vi "AoA Detection 1st TX Ref Signal.vi"() -> ()   [LabVIEW 2015]
doc: "Continuously generates a communication signal that starts immediately. The device is not synchronized to external reference clocks or time bases."
uses:
  <instrlib>/niUSRP/niUSRP Write Tx Data (CDB Cluster).vi
  <vilib>/measure/NI_MABase.lvlib
panel:
  out "TX1":bool
  out "coerced gain":dbl format="%#_6f"
  in  "active antenna":string="TX1"
  out "coerced carrier frequency":dbl format="%#_6p"
  out "coerced IQ rate":dbl format="%#_6p"
  in  "gain":dbl=10.0 format="%#_6f"
  in  "carrier frequency":dbl=900000000.0 format="%#_6p"
  in  "IQ rate":dbl=1000000.0 format="%#_6p"
  out "TX2":bool
  in  "device names":refnum<k15>="192.168.10.2"
  in  "tone frequency":dbl=10000.0 format="%#_6p"
  out "Waveform Graph":waveform(dbl)[](graph)
  in  "waveform size":dbl=10000.0
  in  "timeout":dbl=10.0
  out "error out":errorcluster
  in  "stop":bool
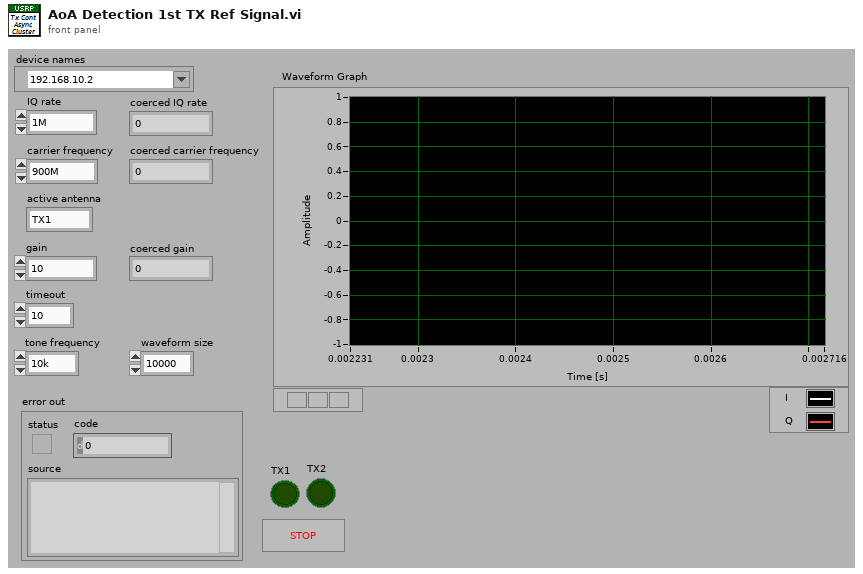
[diagram p1: front panel]
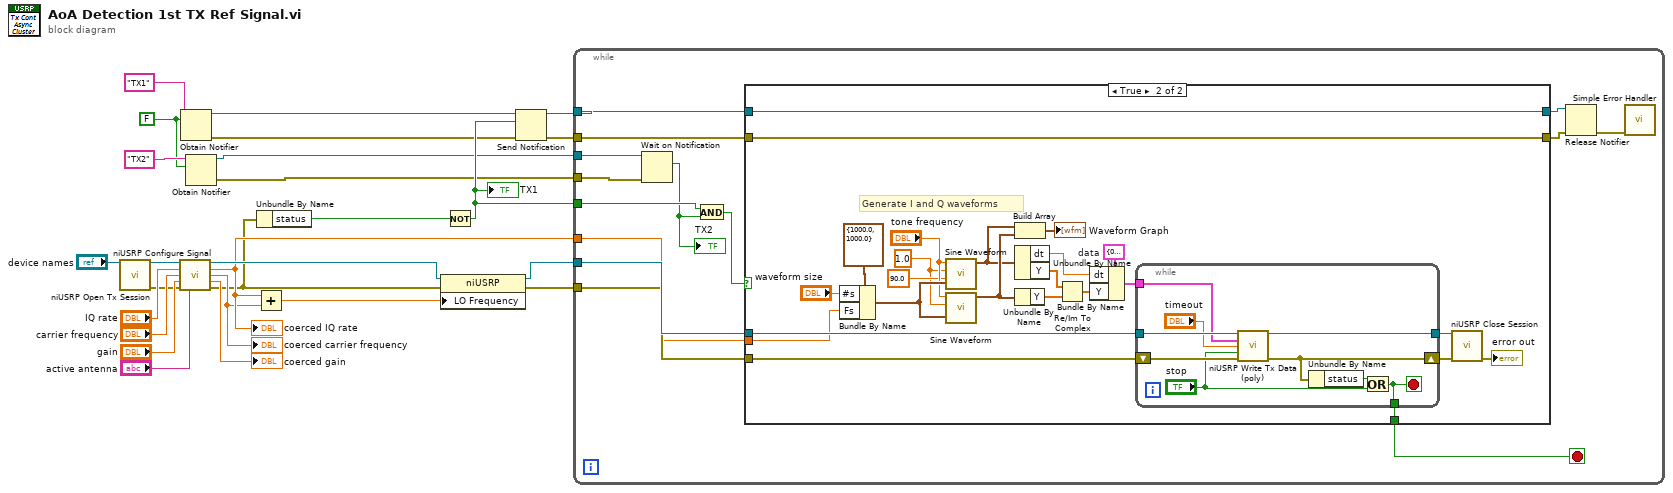
[diagram p0: block diagram]
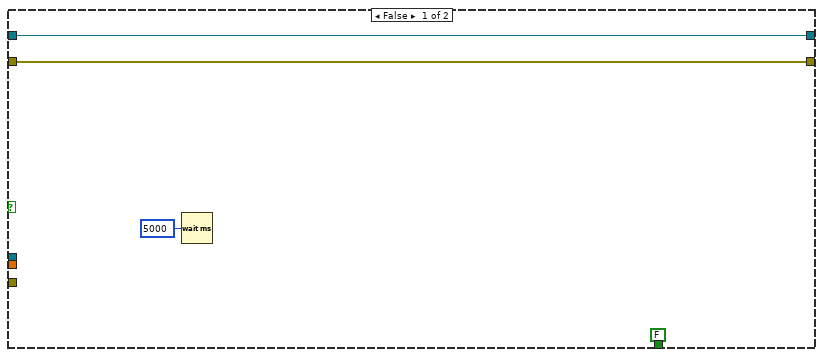
[diagram p2: hidden frame]
diagram:
  w1 = FALSE
  n1 = call <instrlib>:"niUSRP Open Tx Session.vi"("device names"="device names") -> ("session handle out"=w20:refnum<k15>, "error out"=w19:errorcluster)  [unwired: 13 in]
  n2 = call <instrlib>:"niUSRP Configure Signal.vi"("session handle"=w20, "IQ rate"="IQ rate", "carrier frequency"="carrier frequency", "gain"="gain", "error in (no error)"=w19, "active antenna"="active antenna") -> ("session handle out"=w17:refnum<k15>, "coerced IQ rate"=w15:dbl, "coerced carrier frequency"=w14:dbl, "coerced gain"=→"coerced gain":dbl, "error out"=w12:errorcluster)  [unwired: 5 in]
  "coerced IQ rate" <- w15
  "coerced carrier frequency" <- w14
  n3 = Obtain Notifier(name (unnamed)="TX1", notification data type=w1) -> (notifier out=w9:refnum<notifier>, error out=w7:errorcluster)  [unwired: 2 in, 1 out]
  n4 = Obtain Notifier(name (unnamed)="TX2", notification data type=w1) -> (notifier out=w3:refnum<notifier>, error out=w2:errorcluster)  [unwired: 2 in, 1 out]
  n5 = Add(x=w15, y=w14) -> (x+y=w13:dbl)
  n6 = Unbundle By Name(w12) -> ("status"=w18:bool)
  n7 = property class="niUSRP"(reference=w17, error in=w12, "LO Frequency"=w13) -> (reference out=w16:refnum<k15>, error out=w11:errorcluster)
  n8 = Not(x=w18) -> (.not. x?=w8:bool)
  "TX1" <- w8
  n9 = Send Notification(notification=w8, notifier=w9, error in (no error)=w7) -> (notifier out=w6:refnum<notifier>, error out=w5:errorcluster)
  n10 = while {
    tunnel: w16 -> [w39]
    tunnel: w11 -> [w38]
    tunnel: w15 -> [w37]
    tunnel: w8 -> [w35]
    tunnel: w6 -> [w30]
    tunnel: w5 -> [w28]
    tunnel: w3 -> [w33]
    tunnel: w2 -> [w32]
    stop <- w36 stop-if-true
    n11 = Wait on Notification(notifier=w33, error in (no error)=w32) -> (notification=w31:bool)  [unwired: 2 in, 3 out]
    "TX2" <- w31
    n12 = And(x=w35, y=w31) -> (x .and. y?=w40:bool)
    n13 = case shown="True" w40 {
      tunnel: w39 -> [_ w51]
      tunnel: w38 -> [_ w50]
      tunnel: w37 -> [_ w49]
      tunnel: [FALSE w48] -> w36
      tunnel: w30 -> [w42 w46]
      tunnel: [w42 w46] -> w29
      tunnel: w28 -> [w41 w45]
      tunnel: [w41 w45] -> w27
      frame False {
        n14 = Wait (ms)(milliseconds to wait=u32 5000) -> ()  [unwired: 1 out]
      }
      frame True {
        w47 = 1.0 ("amplitude")
        w54 = cluster{"t0":dbl, "dt":dbl, "Y":cdb[]} {"t0"=0.0, "dt"=1.0, "Y"=[]}  # data
        # "Generate I and Q waveforms"
        n15 = Bundle By Name(cluster=cluster{"Fs":dbl, "#s":dbl} {"Fs"=1000.0, "#s"=1000.0} ("sampling info"), "#s"="waveform size", "Fs"=w49) -> (w64:cluster{"Fs":dbl, "#s":dbl})
        n16 = call <vilib>:"Sine Waveform.vi"("sampling info"=w64, "phase"=90.0, "amplitude"=w47, "frequency"="tone frequency") -> ("signal out"=w61:waveform(dbl))  [unwired: 6 in, 1 out]
        n17 = call <vilib>:"Sine Waveform.vi"("sampling info"=w64, "amplitude"=w47, "frequency"="tone frequency") -> ("signal out"=w62:waveform(dbl))  [unwired: 7 in, 1 out]
        n18 = Build Array(w61, w62) -> (→"Waveform Graph":waveform(dbl)[])
        n19 = Unbundle By Name(w61) -> ("dt"=w57:dbl, "Y"=w60:dbl[])
        n20 = Unbundle By Name(w62) -> ("Y"=w59:dbl[])
        n21 = Re/Im To Complex(1:w59, 2:w60) -> (0:w56:cdb[])
        n22 = Bundle By Name(cluster=w54, "dt"=w57, "Y"=w56) -> (w55:cluster{"t0":dbl, "dt":dbl, "Y":cdb[]})
        n23 = while {
          tunnel: w51 -> [w77]
          tunnel: [w74] -> w67
          shift-right: [w73] -> w66
          shift-left: w50 -> [w76]
          tunnel: w55 -> [w72]
          tunnel: [w69] -> w48
          stop <- w69 stop-if-true
          n24 = call-poly <instrlib>:"niUSRP Write Tx Data (poly).vi"("session handle"=w77, "data"=w72, "timeout"="timeout", "end of data?"="stop", "error in (no error)"=w76) -> ("session handle out"=w74:refnum<k15>, "error out"=w73:errorcluster)  [unwired: 9 in]
          n25 = Unbundle By Name(w73) -> ("status"=w71:bool)
          n26 = Or(x=w71, y="stop") -> (x .or. y?=w69:bool)
        }
        n27 = call <instrlib>:"niUSRP Close Session.vi"("session handle"=w67, "error in (no error)"=w66) -> ("error out"=→"error out":errorcluster)  [unwired: 13 in]
      }
    }
    n28 = Release Notifier(notifier=w29, error in (no error)=w27) -> (error out=w34:errorcluster)  [unwired: 1 in, 2 out]
    n29 = call <vilib>:"Simple Error Handler.vi"("error in (no error)"=w34) -> ()  [unwired: 4 in, 5 out]
  }
